vi "Read.vi"(11 "LowLimit Condition Config in":refnum<class "LowLimit Condition Config.lvclass">) -> (2 "Limit":dbl, 3 "Source":string)   [LabVIEW 2020, in "VolatusSeqConfig.lvlib" / "LowLimit Condition Config.lvclass"]
uses:
  LowLimit Condition Config.lvclass
  LowLimit Condition Config.lvclass/LowLimit Condition Config.ctl
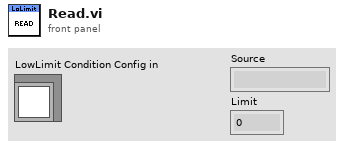
[diagram p1: front panel]
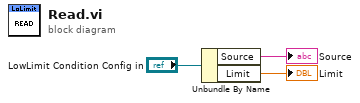
[diagram p0: block diagram]
diagram:
  n1 = Unbundle By Name("LowLimit Condition Config in") -> ("Source"=→"Source":string, "Limit"=→"Limit":dbl)
